vi "PIM Strip Chart Details.vi"(0 "Update Rate":u8(ring) items=["Fastest", "1", "2", "5", "10", "15"]) -> (1 "Seconds per Point":dbl, 2 "Strip Span, seconds":dbl)   [LabVIEW 2011]
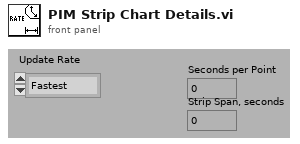
[diagram p1: front panel]
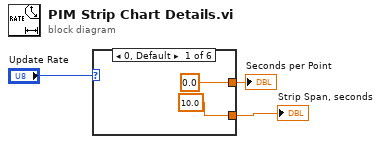
[diagram p0: block diagram]
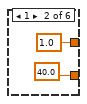
[diagram p2: hidden frame]
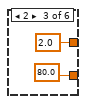
[diagram p3: hidden frame]
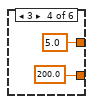
[diagram p4: hidden frame]
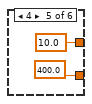
[diagram p5: hidden frame]
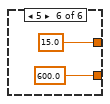
[diagram p6: hidden frame]
diagram:
  n1 = case shown="0, Default" "Update Rate" {
    tunnel: [0.0 1.0 2.0 5.0 10.0 15.0] -> w2
    tunnel: [10.0 40.0 80.0 200.0 400.0 600.0] -> w1
    frame 0, Default {
    }
    frame 1 {
    }
    frame 2 {
    }
    frame 3 {
    }
    frame 4 {
    }
    frame 5 {
    }
  }
  "Seconds per Point" <- w2
  "Strip Span, seconds" <- w1
